vi "Init_All_AE.vi"(7 "Flat File Path":path=path "C:/Users/STED/Desktop/Cambridge STED Control Software/Host VIs/SLM/Flatness Correction LSH0700935/CAL_LSH0700935_770nm.bmp", 8 "HoloArray In":T1[](array[typedef]) {"Modes"."Amplititute" step=0.05}, 11 "General settings":T2={"Holo size (pixels)"=300, "Top hat radius"=0.5, "Number of modes"=20, "Bkg gradient X"=-40.0, "Bkg gradient Y"=-40.0, "Flat"=FALSE, "Mode Matrix"=0}) -> (0 "Holo Array Out":T1[](array[typedef]) {"Modes"."Amplititute" step=0.05})   [LabVIEW 2014]
uses:
  Controls/Holo Controls.ctl
  Controls/SLM General Settings.ctl
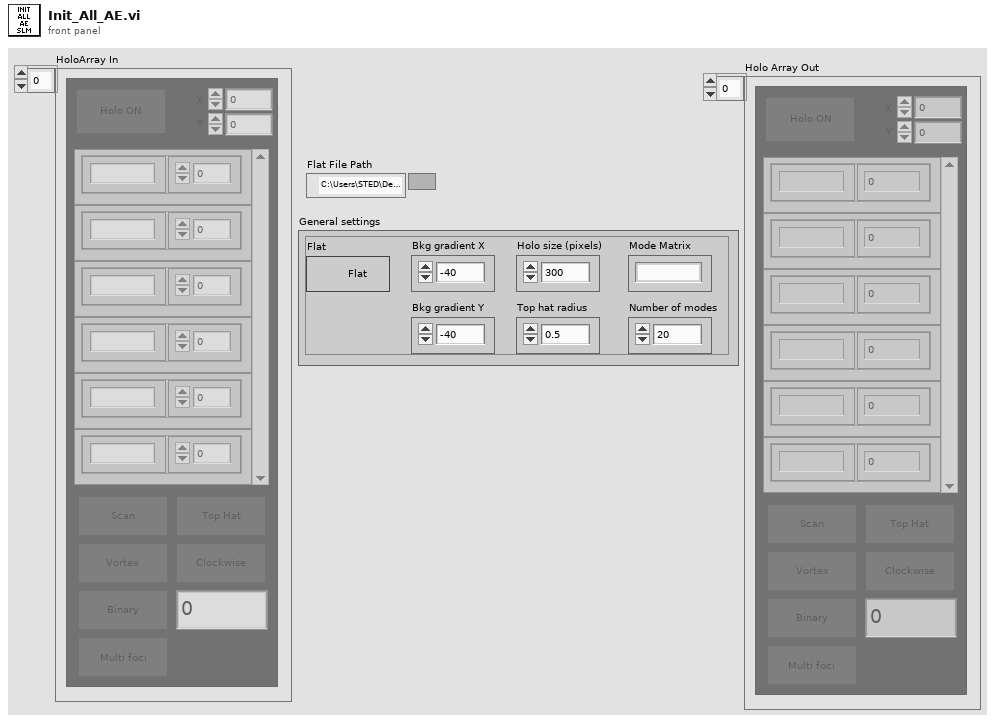
[diagram p1: front panel]
types:
  T1 = typedef "Holo Controls.ctl" = cluster{"Top Hat":bool, "Modes":cluster{"Mode ID":string, "Amplititute":dbl}[], "Vortex":bool, "Clockwise":bool, "X":dbl, "Y":dbl, "Holo ON":bool, "Scan":bool, "Binary":bool, "Binary Angle":dbl, "Multi foci":bool}
  T2 = typedef "SLM General Settings.ctl" = cluster{"Holo size (pixels)":i32, "Top hat radius":dbl, "Number of modes":i32, "Bkg gradient X":dbl, "Bkg gradient Y":dbl, "Flat":bool, "Mode Matrix":u16}
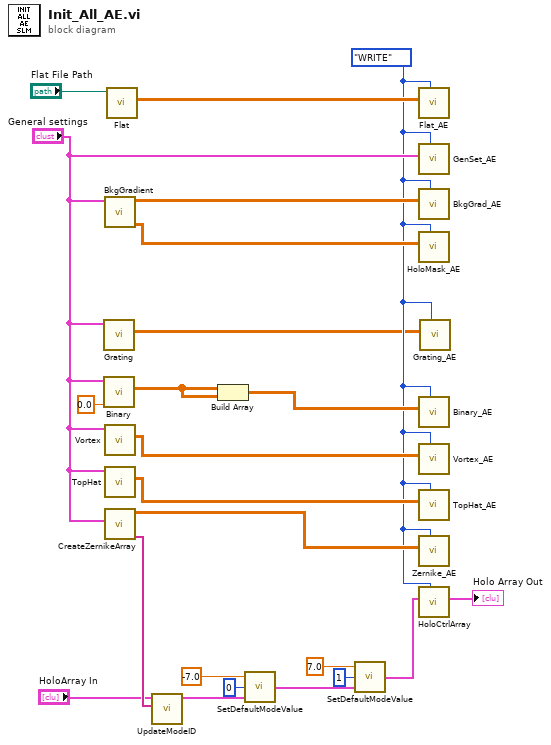
[diagram p0: block diagram]
diagram:
  w2 = enum16{"READ", "WRITE"}."WRITE" ("Action")
  n1 = call "Grating.vi"("General settings"="General settings") -> ("grating"=w1:dbl[][])  [unwired: 10 in]
  n2 = call "Binary.vi"("Angle"=0.0, "General settings"="General settings") -> ("Binary"=w5:dbl[][])  [unwired: 9 in]
  n3 = call "BkgGradient.vi"("General settings"="General settings") -> ("Holo mask"=w16:dbl[][], "gradient"=w15:dbl[][])  [unwired: 9 in]
  n4 = call "Vortex.vi"("General settings"="General settings") -> ("Vortex"=w20:dbl[][])  [unwired: 10 in]
  n5 = call "TopHat.vi"("General settings"="General settings") -> ("TopHat"=w19:dbl[][])  [unwired: 10 in]
  n6 = call "CreateZernikeArray.vi"("General settings"="General settings") -> ("Mode IDs"=w17:string[], "Modes Out"=w18:dbl[][][])  [unwired: 9 in]
  n7 = call "Flat.vi"("File Path"="Flat File Path") -> ("Flatness"=w23:dbl[][])  [unwired: 10 in]
  n8 = call "UpdateModeID.vi"("Mode IDs"=w17, "Array in"="HoloArray In") -> ("Array out"=w14:T1[])  [unwired: 9 in]
  n9 = Build Array(w5, w5) -> (w4:dbl[][][])
  n10 = call "SetDefaultModeValue.vi"("Array in"=w14, "index"=0, "Amplititute"=-7.0) -> ("output array"=w11:T1[])
  n11 = call "SetDefaultModeValue.vi"("Array in"=w11, "index"=1, "Amplititute"=7.0) -> ("output array"=w8:T1[])
  n12 = call "Flat_AE.vi"("Action"=w2, "Flat In"=w23) -> ()  [unwired: 9 in, 1 out]
  n13 = call "GenSet_AE.vi"("Enum"=w2, "General settings"="General settings") -> ()  [unwired: 9 in, 1 out]
  n14 = call "BkgGrad_AE.vi"("Action"=w2, "BkgGrad In"=w15) -> ()  [unwired: 9 in, 1 out]
  n15 = call "HoloMask_AE.vi"("Action"=w2, "HoloMask In"=w16) -> ()  [unwired: 9 in, 1 out]
  n16 = call "Binary_AE.vi"("Action"=w2, "BINARY In"=w4) -> ()  [unwired: 9 in, 1 out]
  n17 = call "Vortex_AE.vi"("Action"=w2, "Vortex In"=w20) -> ()  [unwired: 9 in, 1 out]
  n18 = call "TopHat_AE.vi"("Action"=w2, "TopHat In"=w19) -> ()  [unwired: 9 in, 1 out]
  n19 = call "Zernike_AE.vi"("Action"=w2, "Zernike In"=w18) -> ()  [unwired: 9 in, 1 out]
  n20 = call "HoloCtrlArray.vi"("Action"=w2, "Holo Array In"=w8) -> ("Holo Array Out"=→"Holo Array Out":T1[])  [unwired: 9 in]
  n21 = call "Grating_AE.vi"("Action"=w2, "Grating In"=w1) -> ()  [unwired: 9 in, 1 out]
